vi "Is Door Open.vi"(0 "Interface_object in":refnum<class "DoorInterface.lvclass">, 5 "error in (no error)":errorcluster) -> (14 "Interface_object out":refnum<class "DoorInterface.lvclass">, 16 "Is Door Open?":bool, 19 "error out":errorcluster)   [LabVIEW 2018, in "DoorInterface.lvclass"]
doc: "AZ Interface method template"
uses:
  DoorInterface.lvclass
  DoorInterface.lvclass/DoorInterface.ctl
panel:
  # "Add terminals, connect them to terminal pattern,\nand save the method.\n\nDo not edit BD of this method"
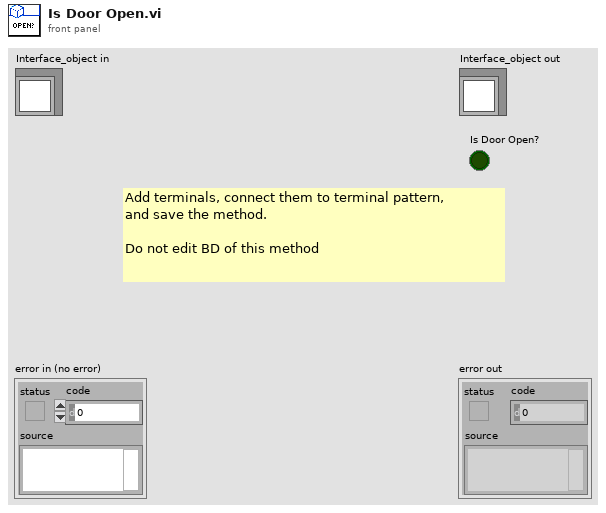
[diagram p1: front panel]
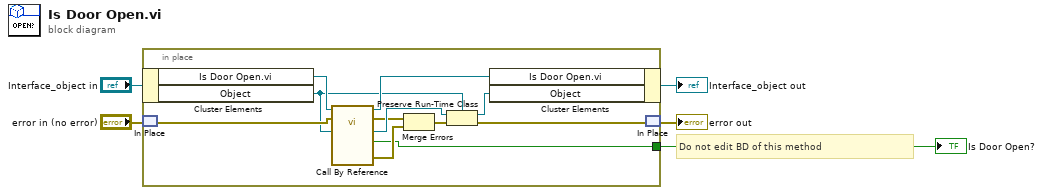
[diagram p0: block diagram]
diagram:
  # "Do not edit BD of this method"
  n1 = in-place {
    in-place-border: [w6] -> w1
    n2 = in-place-cluster #1("Interface_object in") -> ("Is Door Open.vi"=w16:refnum<vi>, "Object"=w9:refnum<class>)
    n3 = in-place-match #2("error in (no error)") -> (w13:errorcluster)
    n4 = call-by-ref "?"(reference=w16, error in=w13, "Interface_object in"=w9) -> (reference out=w15:refnum<vi>, error out=w11:errorcluster, "Interface_object out"=w14:refnum<class>, "Is Door Open?"=w6:bool, 19:"error out"=w12:errorcluster)  [unwired: 16 in]
    n5 = Merge Errors(w11, w12) -> (w8:errorcluster)
    n6 = Preserve Run-Time Class(object in=w14, error in=w8, 2:w9) -> (object out=w10:refnum<class>, error out=w7:errorcluster)
    n7 = in-place-cluster #1("Is Door Open.vi"=w15, "Object"=w10) -> (→"Interface_object out":refnum<class "DoorInterface.lvclass">)
    n8 = in-place-match #2(w7) -> (→"error out":errorcluster)
  }
  "Is Door Open?" <- w1
